vi "Agilent 3458 Acquire Statistics Measurement.vi"() -> ()   [LabVIEW 2020, in "3458A Virtual Digitizer.lvlib" / "3458A Basic Driver.lvlib"]
doc: "Shows how to configure and take measurements and then display a statistical analysis of these measurements."
uses:
  3458A Basic Driver.lvlib
  Public/Data/Read Measurement(Math).vi
panel:
  in  "Manual Range (1.00)":dbl=1.0 format="%_3g"
  out "Minimum":dbl
  out "Standard Deviation":dbl
  out "Average":dbl
  out "Count":dbl
  out "Maximum":dbl
  in  "Maximum Time (10000ms)":u32=10000
  in  "Trigger Count (1)":dbl=1.0 format="%#.6g"
  in  "Sample Count (1)":dbl=10.0 format="%#.6g"
  in  "Trigger Type (0:Auto)":u16(ring) items=["Auto", "External", "Level", "Line", "Synchronous"]
  in  "Auto Range (1:ON)":u16(ring)=1 items=["OFF", "ON", "ONCE"]
  in  "Frequency Source (3: AC Voltage)":u16(ring)=3 items=["AC + DC Current", "AC + DC Voltage", "AC Current", "AC Voltage"]
  in  "Manual Resolution (2: 6.5 digits)":enum16{"4.5", "5.5", "6.5", "7.5", "8.5"}(ring)=enum."6.5"
  in  "Function (0: DC Voltage)":u16(ring) items=["DC Voltage", "AC Voltage", "AC + DC Voltage", "DC Current", "AC Current", "AC + DC Current", "2-Wire Resistance", "4-Wire Resistance", "Frequency", "Period", "Direct Sampling DC", "Direct Sampling AC"]
  in  "VISA resource name":refnum<visa-resource-name>
  # "(c) 2007  National Instruments.  ALL RIGHTS RESERVED."
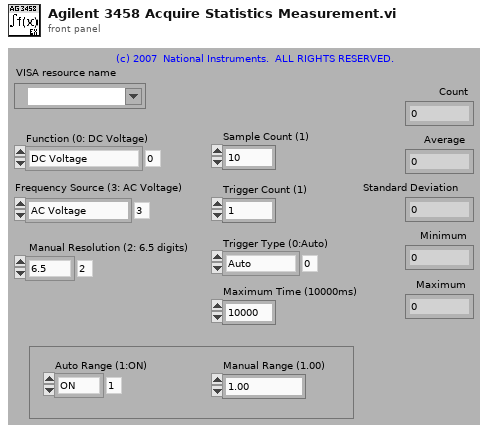
[diagram p1: front panel]
types:
  T1 = enum16{"CRTD85", "CRTD92", "CTHRM", "CTHRM2K", "CTHRM10K", "dB", "dBm", "Filter", "FRTD85", "FRTD92", "FTHRM", "FTHRM2K", "FTHRM10K", "None", "Null", "Pass/Fail", "Percent", "RMS", "Scale", "Statistics"}
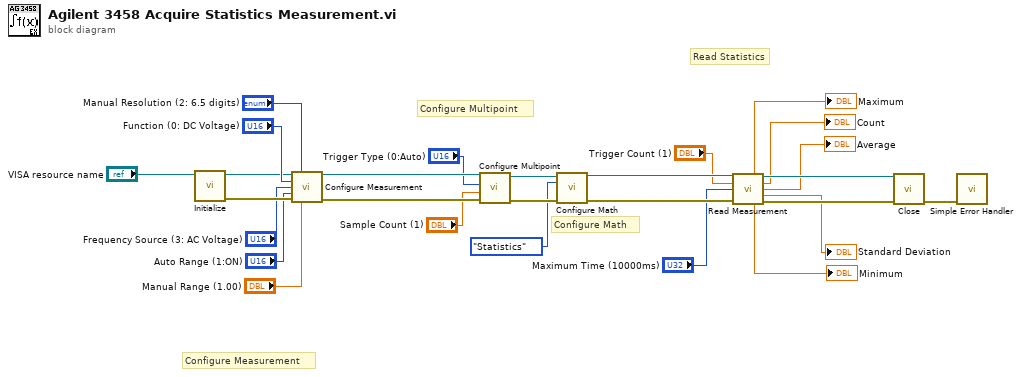
[diagram p0: block diagram]
diagram:
  # "Configure Multipoint"
  # "Read Statistics"
  # "Configure Math"
  # "Configure Measurement"
  n1 = call "Initialize.vi"("VISA resource name"="VISA resource name") -> ("error out"=w15:errorcluster, "VISA resource name out"=w16:refnum<visa-resource-name>)  [unwired: 8 in, 1 out]
  n2 = call "Configure Measurement.vi"("VISA resource name"=w16, "Manual Resolution (2: 6.5 digits)"="Manual Resolution (2: 6.5 digits)", "Function (0: DC Voltage)"="Function (0: DC Voltage)", "Frequency Source (3: AC Voltage)"="Frequency Source (3: AC Voltage)", "Auto Range (1:ON)"="Auto Range (1:ON)", "error in (no error)"=w15, "Manual Range (1.00)"="Manual Range (1.00)") -> ("VISA resource name out"=w20:refnum<visa-resource-name>, "error out"=w19:errorcluster)  [unwired: 7 in]
  n3 = call "Configure Multipoint.vi"("error in (no error)"=w19, "Sample Count (1)"="Sample Count (1)", "Trigger Type (0:Auto)"="Trigger Type (0:Auto)", "VISA resource name"=w20) -> ("error out"=w17:errorcluster, "VISA resource name out"=w18:refnum<visa-resource-name>)  [unwired: 6 in]
  n4 = call "Configure Math.vi"("VISA resource name"=w18, "Operation (13:None)"=T1."Statistics", "error in (no error)"=w17) -> ("VISA resource name out"=w27:refnum<visa-resource-name>, "error out"=w26:errorcluster)  [unwired: 11 in]
  n5 = call-poly "Read Measurement.vi"("VISA resource name"=w27, "Trigger Count (1)"="Trigger Count (1)", "Maximum Time (10000ms)"="Maximum Time (10000ms)", "error in (no error)"=w26) -> ("Maximum"=→"Maximum":dbl, "VISA resource name out"=w24:refnum<visa-resource-name>, "Count"=→"Count":dbl, "Average"=→"Average":dbl, "Standard Deviation"=→"Standard Deviation":dbl, "Minimum"=→"Minimum":dbl, "error out"=w23:errorcluster)  [unwired: 5 in]
  n6 = call "Close.vi"("error in (no error)"=w23, "VISA resource name"=w24) -> ("error out"=w25:errorcluster)  [unwired: 9 in]
  n7 = call <vilib>:"Simple Error Handler.vi"("error in (no error)"=w25) -> ()  [unwired: 4 in, 5 out]
